vi "CalculateQuatWithRatios.vi"(8 "FloatRatioB":dbl, 9 "qb (in)":T1, 10 "FloatRatioA":dbl, 11 "qa (in)":T1) -> (3 "Quat (out)":T1)   [LabVIEW 2016]
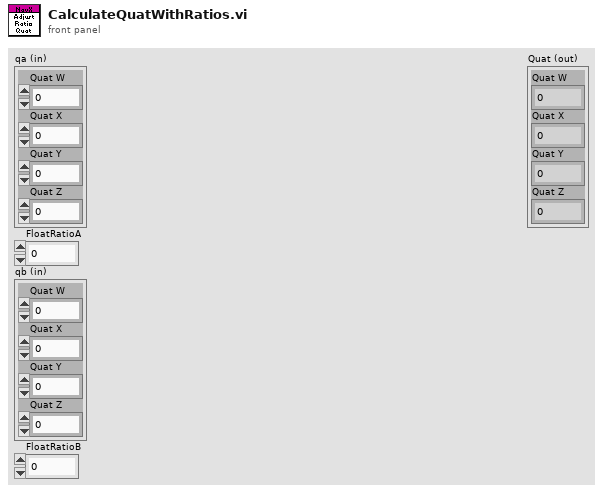
[diagram p1: front panel]
types:
  T1 = cluster{"Quat W":dbl, "Quat X":dbl, "Quat Y":dbl, "Quat Z":dbl}
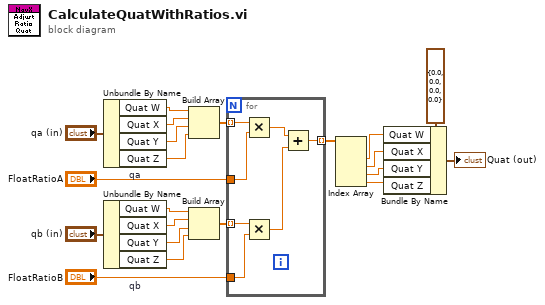
[diagram p0: block diagram]
diagram:
  n1 = Unbundle By Name "qa"("qa (in)") -> ("Quat W"=w12:dbl, "Quat X"=w13:dbl, "Quat Y"=w14:dbl, "Quat Z"=w15:dbl)
  n2 = Unbundle By Name "qb"("qb (in)") -> ("Quat W"=w16:dbl, "Quat X"=w17:dbl, "Quat Y"=w18:dbl, "Quat Z"=w19:dbl)
  n3 = Build Array(w12, w13, w14, w15) -> (w20:dbl[])
  n4 = Build Array(w16, w17, w18, w19) -> (w21:dbl[])
  n5 = for {
    tunnel: w20 -> [w28] mode=indexing
    tunnel: w21 -> [w27] mode=indexing
    tunnel: [w24] -> w8 mode=indexing
    tunnel: "FloatRatioA" -> [w22]
    tunnel: "FloatRatioB" -> [w23]
    n6 = Multiply(x=w28, y=w22) -> (x*y=w26:dbl)
    n7 = Multiply(x=w27, y=w23) -> (x*y=w25:dbl)
    n8 = Add(x=w26, y=w25) -> (x+y=w24:dbl)
  }
  n9 = Index Array(array=w8) -> (element #1=w7:dbl, element #2=w6:dbl, element #3=w4:dbl, element #4=w5:dbl)  [unwired: 4 in]
  n10 = Bundle By Name(cluster=T1 {"Quat W"=0.0, "Quat X"=0.0, "Quat Y"=0.0, "Quat Z"=0.0} ("Quat (out)"), "Quat W"=w7, "Quat X"=w6, "Quat Y"=w4, "Quat Z"=w5) -> (→"Quat (out)":T1)
